vi "Match Initiate Upload Response.vi"(8 "error in":errorcluster, 10 "Frame Data":u8[](array[numeric]), 11 "SDO Transfer in":refnum<class "SDO Transfer.lvclass">) -> (0 "error out":errorcluster, 2 "Match":bool, 3 "SDO Transfer out":refnum<class "SDO Transfer.lvclass">)   [LabVIEW 2020, in "CANopen.lvlib" / "SDO Manager.lvlib" / "Upload Transfer.lvclass"]
uses:
  Upload Transfer.lvclass
  SDO Transfer/SDO Transfer.lvclass
  Segmented Upload Transfer/Segmented Upload Transfer.lvclass
  HAL/Source/Interfaces/ICommunicate/ICommunicate.lvclass
  Upload Transfer.lvclass/Upload Transfer.ctl
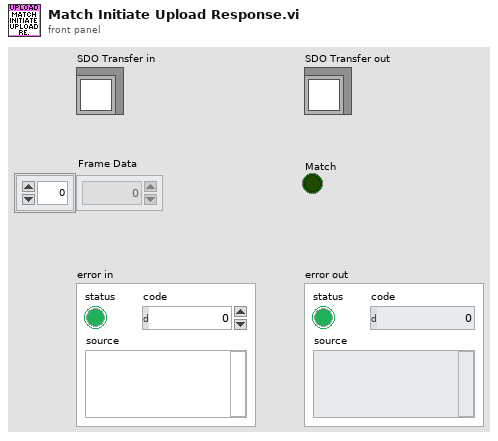
[diagram p1: front panel]
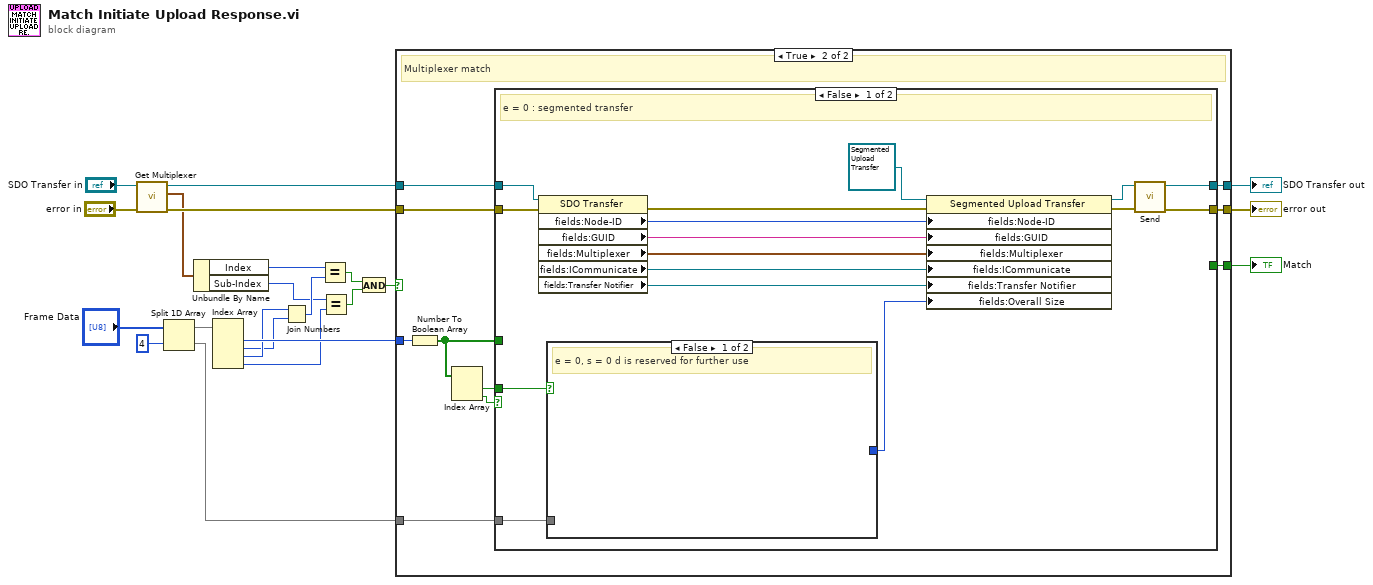
[diagram p0: block diagram]
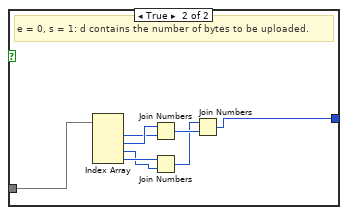
[diagram p3: hidden frame]
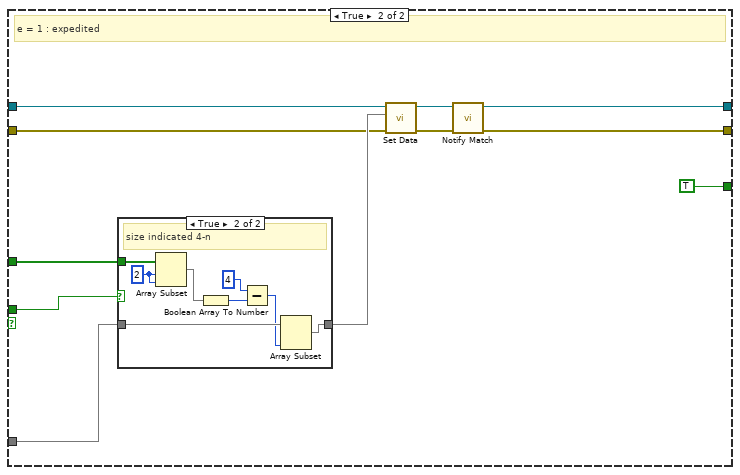
[diagram p4: hidden frame]
diagram:
  n1 = call "Get Multiplexer.vi"("error in"="error in", "SDO Transfer in"="SDO Transfer in") -> ("error out"=w13:errorcluster, "Multiplexer"=w8:cluster{"Index":u16, "Sub-Index":u8}, "SDO Transfer out"=w12:refnum<class "SDO Transfer.lvclass">)  [unwired: 7 in]
  n2 = Split 1D Array(array="Frame Data", index=4) -> (first subarray=w16:u8[], second subarray=w7:u8[])
  n3 = Unbundle By Name(w8) -> ("Index"=w11:u16, "Sub-Index"=w9:u8)
  n4 = Index Array(array=w16) -> (element #1=w14:u8, element #2=w1:u8, element #3=w2:u8, element #4=w3:u8)  [unwired: 4 in]
  n5 = Join Numbers(hi=w2, lo=w1) -> ((hi.lo)=w10:u16)
  n6 = Equal?(x=w11, y=w10) -> (x = y?=w5:bool)
  n7 = Equal?(x=w9, y=w3) -> (x = y?=w4:bool)
  n8 = And(x=w5, y=w4) -> (x .and. y?=w6:bool)
  n9 = case shown="True" w6 {
    tunnel: [_ w31] -> w22
    tunnel: [w23 w30] -> w21
    tunnel: [w24 w29] -> w19
    tunnel: w14 -> [_ w28]
    tunnel: w13 -> [w24 w27]
    tunnel: w12 -> [w23 w26]
    tunnel: w7 -> [_ w25]
    frame False {
      # "Multiplexer mismatch"
    }
    frame True {
      # "Multiplexer match"
      n10 = Number To Boolean Array(number=w28) -> (Boolean array=w32:bool[])
      n11 = Index Array(array=w32) -> (element #1=w34:bool, element #2=w33:bool)  [unwired: 2 in]
      n12 = case shown="False" w33 {
        tunnel: [w43 w69] -> w29
        tunnel: w26 -> [w50 w61]
        tunnel: [w42 w68] -> w30
        tunnel: [_ TRUE] -> w31
        tunnel: w25 -> [w48 w65]
        tunnel: w34 -> [w49 w64]
        tunnel: w32 -> [_ w63]
        tunnel: w27 -> [w35 w62]
        frame False {
          # "e = 0 : segmented transfer"
          n13 = property class="SDO Transfer"(reference=w50, error in=w35) -> (error out=w46:errorcluster, "fields:Node-ID"=w38:u8, "fields:GUID"=w36:string, "fields:Multiplexer"=w39:cluster{"Index":u16, "Sub-Index":u8}, "fields:ICommunicate"=w40:refnum<class "ICommunicate.lvclass">, "fields:Transfer Notifier"=w41:refnum<notifier>)  [unwired: 1 out]
          n14 = case shown="False" w49 {
            tunnel: w48 -> [_ w58]
            tunnel: [_ w51] -> w37
            frame False {
              # "e = 0, s = 0 d is reserved for further use"
            }
            frame True {
              # "e = 0, s = 1: d contains the number of bytes to be uploaded."
              n15 = Index Array(array=w58) -> (element #1=w54:u8, element #2=w55:u8, element #3=w56:u8, element #4=w57:u8)  [unwired: 4 in]
              n16 = Join Numbers(hi=w55, lo=w54) -> ((hi.lo)=w53:u16)
              n17 = Join Numbers(hi=w57, lo=w56) -> ((hi.lo)=w52:u16)
              n18 = Join Numbers(hi=w52, lo=w53) -> ((hi.lo)=w51:u32)
            }
          }
          n19 = property class="Segmented Upload Transfer"(reference=refnum<class "Segmented Upload Transfer.lvclass"> refnum ("CANopen Master:Segmented Upload Transfer.lvclass"), error in=w46, "fields:Node-ID"=w38, "fields:GUID"=w36, "fields:Multiplexer"=w39, "fields:ICommunicate"=w40, "fields:Transfer Notifier"=w41, "fields:Overall Size"=w37) -> (reference out=w44:refnum<class "Segmented Upload Transfer.lvclass">, error out=w45:errorcluster)
          n20 = call-dynamic "Send.vi"("error in"=w45, "Segmented Upload Transfer"=w44) -> ("error out"=w43:errorcluster, "Segmented Upload Transfer"=w42:refnum<class "Segmented Upload Transfer.lvclass">)  [unwired: 8 in]
        }
        frame True {
          # "e = 1 : expedited"
          n21 = case shown="True" w64 {
            tunnel: [w70 w77] -> w67
            tunnel: w65 -> [w70 w78]
            tunnel: w63 -> [_ w74]
            frame False {
              (unwired) TRUE
              # "size not specified"
            }
            frame True {
              w73 = 2 ("index")
              # "size indicated 4-n"
              n22 = Array Subset(array=w74, index=w73, length=w73) -> (w71:bool[])
              n23 = Boolean Array To Number(Boolean array=w71) -> (number=w72:u32)
              n24 = Subtract(x=u32 4, y=w72) -> (x-y=w76:u32)
              n25 = Array Subset(array=w78, length=w76) -> (w77:u8[])  [unwired: 1 in]
            }
          }
          n26 = call "Set Data.vi"("error in"=w62, "Data"=w67, "SDO Transfer in"=w61) -> ("error out"=w60:errorcluster, "SDO Transfer out"=w59:refnum<class "SDO Transfer.lvclass">)  [unwired: 7 in]
          n27 = call "Notify Match.vi"("error in"=w60, "SDO Transfer in"=w59) -> ("error out"=w69:errorcluster, "SDO Transfer out"=w68:refnum<class "SDO Transfer.lvclass">)  [unwired: 8 in]
        }
      }
    }
  }
  "Match" <- w22
  "SDO Transfer out" <- w21
  "error out" <- w19
